vi "Init.vi"(10 "Error":errorcluster) -> (3 "Merge Error Msg Strategy out":refnum<class "Merge Error Msg Strategy.lvclass">)   [LabVIEW 2021, in "Merge Error Msg Strategy.lvlib" / "Merge Error Msg Strategy.lvclass"]
uses:
  Merge Error Msg Strategy.lvclass
  Merge Error Msg Strategy.lvclass/Merge Error Msg Strategy.ctl
  jettl/Sender/Sender.lvlib
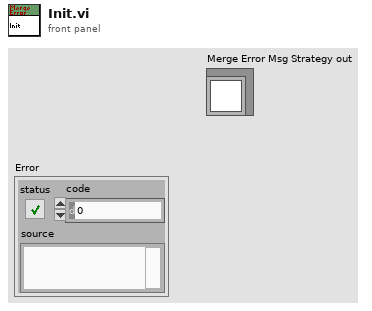
[diagram p1: front panel]
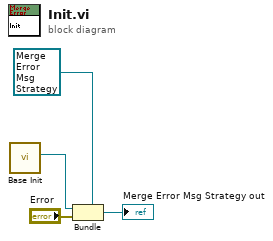
[diagram p0: block diagram]
diagram:
  n1 = call "Base Init.vi"() -> ("Sender"=w1:refnum<class "Sender.lvclass">)  [unwired: 11 in]
  n2 = Bundle "Bundle"(cluster=refnum<class "Merge Error Msg Strategy.lvclass"> refnum ("Merge Error Msg Strategy out"), w1, "Error") -> (→"Merge Error Msg Strategy out":refnum<class "Merge Error Msg Strategy.lvclass">)
